vi "get Moveable.vi"(8 "error in (no error)":errorcluster, 11 "xceDataNode in":refnum<class "xceDataNode.lvclass">) -> (0 "error out":errorcluster, 2 "Moveable":bool, 3 "xceDataNode out":refnum<class "xceDataNode.lvclass">)   [LabVIEW 2013, in "xceDataNode.lvclass"]
doc: "Get Moveable. Gets is a node is moveable, aka drag/dropable and rearrangable in a subNode array."
uses:
  xceDataNode.lvclass
  xceDataNode.lvclass/xceDataNode.ctl
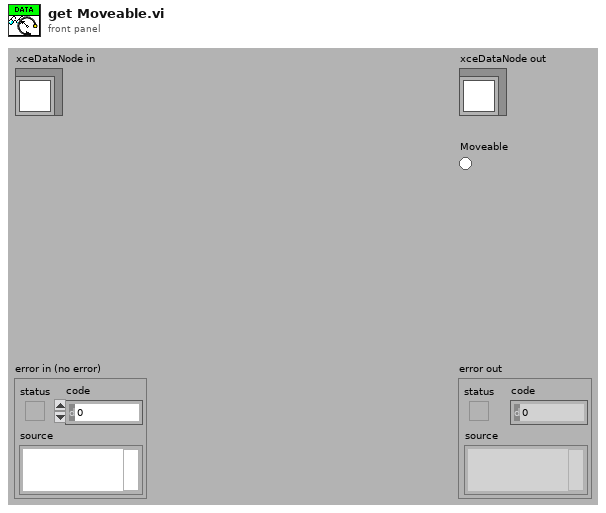
[diagram p1: front panel]
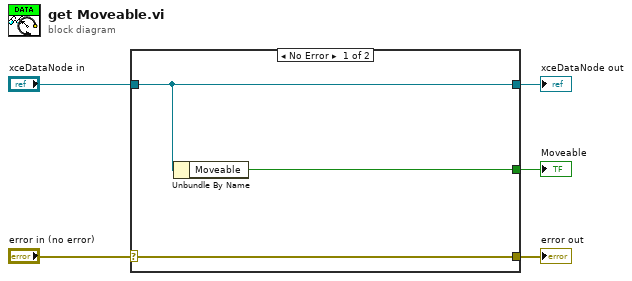
[diagram p0: block diagram]
diagram:
  n1 = case shown="No Error" "error in (no error)" {
    selector: "error in (no error)" -> [w8 w9]
    tunnel: [w8 w9] -> w4
    tunnel: [w7 w10] -> w2
    tunnel: "xceDataNode in" -> [w7 w10]
    tunnel: [w6 _] -> w1
    frame No Error {
      n2 = Unbundle By Name(w7) -> ("Moveable"=w6:bool)
    }
    frame Error {
    }
  }
  "error out" <- w4
  "xceDataNode out" <- w2
  "Moveable" <- w1
